vi "Accel Code Archived 7-29-15.vi"() -> ()   [LabVIEW 2015]
uses:
  <vilib>/rvi/Emulation/niFpgaGetClockAttributes.vi
  <vilib>/rvi/Emulation/niFpgaSctlEmulationGetInTimedLoop.vi
  <vilib>/rvi/Emulation/niFpgaEmulationReportErrorSimple.vi
  FPGA Globals.vi
  <vilib>/rvi/Emulation/niFpgaCriticalErrorInLSC.vi
  <vilib>/IEDriver/SPIandI2C/FPGA/Library/IP SPI&I2C.lvlib
panel:
  out "gXSBRIO":fxp<+/-,32,10>
  out "gYSBRIO":fxp<+/-,32,10>
  out "gZSBRIO":fxp<+/-,32,10>
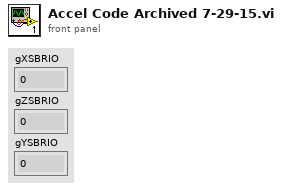
[diagram p1: front panel]
types:
  T1 = cluster{"SCLK":refnum<k21>, "MISO":refnum<k21>, "MOSI":refnum<k21>, "CS 0":refnum<k21>, "CS 1":refnum<k21>, "CS 2":refnum<k21>, "CS 3":refnum<k21>, "CS 4":refnum<k21>, "CS 5":refnum<k21>, "CS 6":refnum<k21>, "CS 7":refnum<k21>, "CS 8":refnum<k21>, "CS 9":refnum<k21>}
  T2 = typedef "IP SPI&I2C.lvlib/Private Data (SPI).ctl" = cluster{"Arm Trigger":refnum<k21>, "API to IP Data":refnum<k21>, "IP to API Data":refnum<k21>, "Configure Register":refnum<k21>, "Configuration Lock":refnum<k21>}
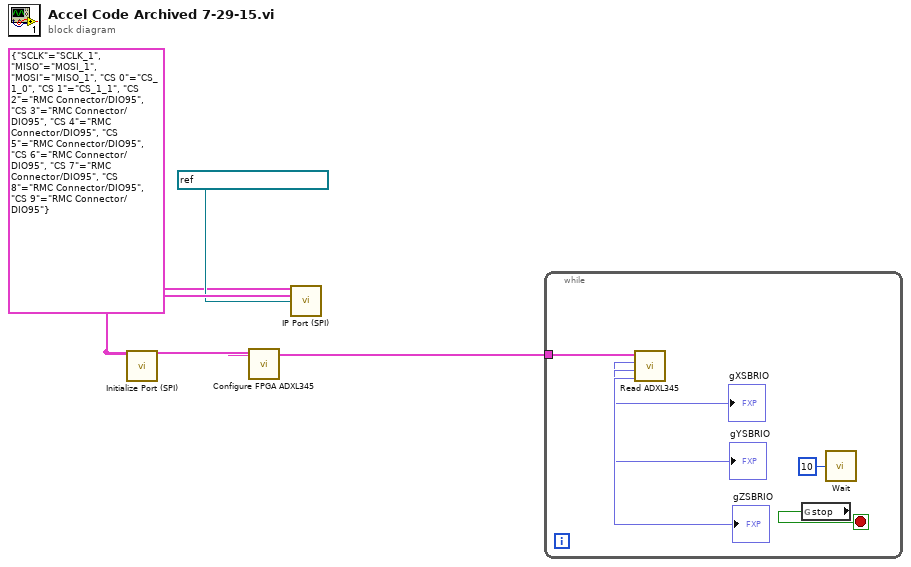
[diagram p0: block diagram]
diagram:
  n1 = call <vilib>:"Initialize Port (SPI).vi"() -> ("Private Data Out"=w2:T2)  [unwired: 14 in, 1 out]
  n2 = call "Configure FPGA ADXL345.vi"("Private Data In"=w2) -> ("Private Data Out"=w1:T2)  [unwired: 10 in]
  n3 = call <vilib>:"IP Port (SPI).vi"("Private Data In"=w2, "SPI FPGA IO"=T1 {"SCLK"="SCLK_1", "MISO"="MOSI_1", "MOSI"="MISO_1", "CS 0"="CS_1_0", "CS 1"="CS_1_1", "CS 2"="RMC Connector/DIO95", "CS 3"="RMC Connector/DIO95", "CS 4"="RMC Connector/DIO95", "CS 5"="RMC Connector/DIO95", "CS 6"="RMC Connector/DIO95", "CS 7"="RMC Connector/DIO95", "CS 8"="RMC Connector/DIO95", "CS 9"="RMC Connector/DIO95"}, "FPGA Clock"=refnum<k21> "40 MHz Onboard Clock") -> ()  [unwired: 13 in]
  n4 = while {
    tunnel: w1 -> [w9]
    stop <- w10 stop-if-true
    n5 = call "Read ADXL345.vi"("Private Data In"=w9) -> ("Z (g)"=→"gZSBRIO":fxp<+/-,32,10>, "Y (g)"=→"gYSBRIO":fxp<+/-,32,10>, "X (g)"=→"gXSBRIO":fxp<+/-,32,10>)  [unwired: 6 in, 1 out]
    n6 = global read "FPGA Globals.vi" "stop"() -> (w10:bool)
    n7 = call "Wait"("Count(mSec)"=u32 10) -> ()  [unwired: 1 out]
  }
